vi "services.vi"(8 "error in (no error)":errorcluster, 11 "system in":refnum<class "system.lvclass">) -> (0 "error out":errorcluster)   [LabVIEW 2021, in "system.lvclass"]
uses:
  system.lvclass
  system.lvclass/system.ctl
panel:
  # "Container for tertiary services, all services\nmust be registers in system and utilize the system.threading\nclass for lifecycle management"
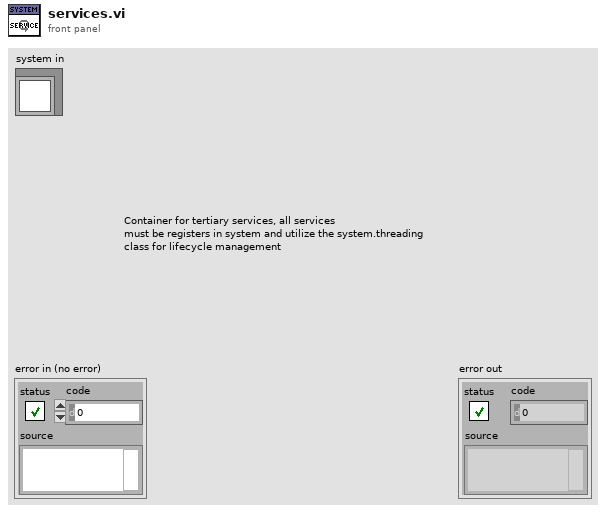
[diagram p1: front panel]
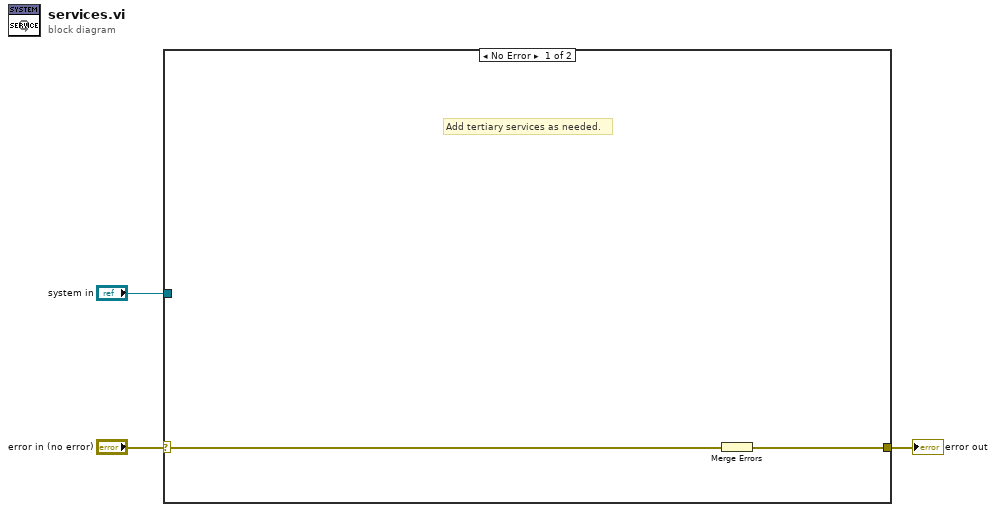
[diagram p0: block diagram]
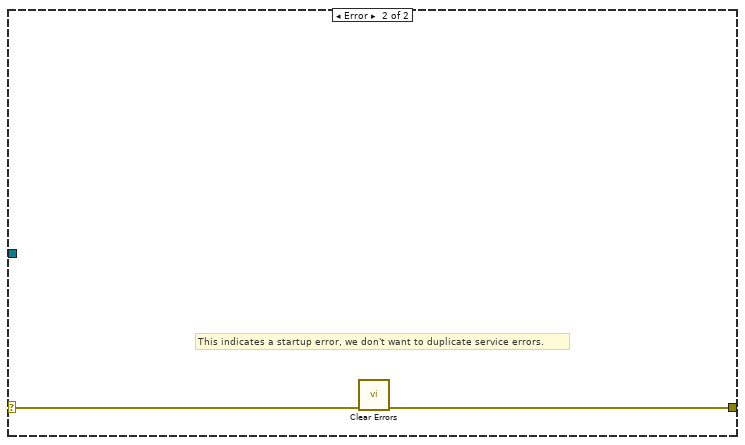
[diagram p2: hidden frame]
diagram:
  n1 = case shown="No Error" "error in (no error)" {
    selector: "error in (no error)" -> [w4 w7]
    tunnel: [w5 w6] -> w2
    tunnel: "system in" -> [_ _]
    frame No Error {
      # "Add tertiary services as needed."
      n2 = Merge Errors(w4) -> (w5:errorcluster)
    }
    frame Error {
      # "This indicates a startup error, we don't want to duplicate service errors."
      n3 = call <vilib>:"Clear Errors.vi"("error in (no error)"=w7) -> ("error out"=w6:errorcluster)  [unwired: 5 in, 1 out]
    }
  }
  "error out" <- w2
